vi "waitNewResults.vi"(8 "error in (no error)":errorcluster, 11 "Instrument.LockinAPI in":refnum<class "Instrument.LockinAPI.lvclass">) -> (0 "error out":errorcluster, 2 "Results (Dictionary)":cluster{"key":string, "value":dbl}[](array[cluster]), 3 "Instrument.LockinAPI out":refnum<class "Instrument.LockinAPI.lvclass">)   [LabVIEW 2019, in "Instrument.LockinAPI.lvclass"]
uses:
  Instrument.LockinAPI.lvclass
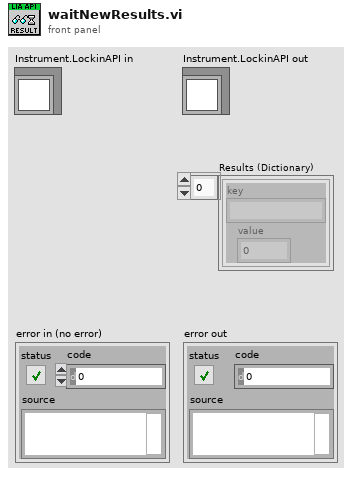
[diagram p1: front panel]
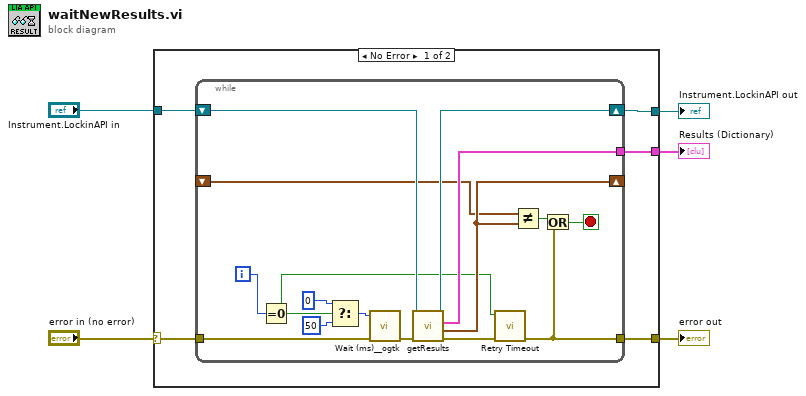
[diagram p0: block diagram]
diagram:
  n1 = case shown="No Error" "error in (no error)" {
    selector: "error in (no error)" -> [w6 w27]
    tunnel: [w10 w27] -> w5
    tunnel: [w9 _] -> w4
    tunnel: "Instrument.LockinAPI in" -> [w8 w28]
    tunnel: [w7 w28] -> w2
    frame No Error {
      n2 = while {
        shift-right: [w24] -> _
        shift-left: _ -> [w12]
        tunnel: w6 -> [w26]
        tunnel: [w15] -> w10
        tunnel: [w13] -> w9
        shift-right: [w22] -> w7
        shift-left: w8 -> [w23]
        i -> [w14]
        stop <- w20 stop-if-true
        n3 = Equal To 0?(x=w14) -> (x = 0?=w11:bool)
        n4 = Select(t=u32 0, s=w11, f=u32 50 ("milliseconds to wait")) -> (s? t:f=w18:u32)
        n5 = call <userlib>:"Wait (ms)__ogtk.vi"("error in (no error)"=w26, "milliseconds to wait"=w18) -> ("error out"=w25:errorcluster)  [unwired: 8 in, 1 out]
        n6 = call-dynamic "getResults.vi"("error in (no error)"=w25, "Instrument.LockinAPI in"=w23) -> ("error out"=w16:errorcluster, "Time Stamp"=w24:timestamp, "Results (Dictionary)"=w13:cluster{"key":string, "value":dbl}[], "Instrument.LockinAPI out"=w22:refnum<class "Instrument.LockinAPI.lvclass">)  [unwired: 6 in]
        n7 = call "Retry Timeout.vi"("error in (no error)"=w16, "reset"=w11) -> ("error out"=w15:errorcluster)  [unwired: 8 in, 1 out]
        n8 = Not Equal?(x=w12, y=w24) -> (x != y?=w21:bool)
        n9 = Or(x=w21, y=w15) -> (x .or. y?=w20:bool)
      }
    }
    frame Error {
    }
  }
  "error out" <- w5
  "Results (Dictionary)" <- w4
  "Instrument.LockinAPI out" <- w2
